vi "USBImageContinuousV1.9.vi"() -> ()   [LabVIEW 2019]
uses:
  atmcd32d.dll
panel:
  in  "Tab Control":T1(tab)
  out "Expected position on spectrometer (pixels):":dbl
  in  "Harmonic":dbl min=10.0 max=40.0
  out "l (nm)":dbl
  out "E (J)":dbl
  out "E (eV)":dbl
  out "Nearest Harmonic of 800nm":dbl
  out "Cursor Position (pixels)":dbl
  out "Distance to nearest harmonic of 800nm (pixels)":dbl
  in  "Grating:":u16(ring) items=["Shimadzu 30-006  "]
  in  "Laser:":u16(ring) items=["800nm  "]
  in  "Trigger":u32(ring) items=["Internal", "External"]
  in  "Exposure Time (secs)":sgl format="%.2f"
  out "Get Acquired Data":u32
  out "Start Acquisition":u32
  out "Detector X Pixels":i32
  out "Detector Y Pixels":i32
  out "Shut Down":u32
  out "Raw Image":i32[][](graph)
  out "Vertical Binned image":i32[](graph)
  out "Get Status":u32
  in  "Stop":bool
  in  "Save Image":bool
  out "Camera Status:":bool
  out "Last Image Saved:":string
  in  "Calibration Date":u16(ring) items=["first calibration - 7/31", "7/31-current"]
  out "Calibration Date: indicator:":u16(ring) items=["first calibration - 7/31", "7/31-current"]
  out "Status":u32
  out "Camera outputs":T2
  out "Camera inputs":T3
  in  "Correct for QE?":bool
  in  "IR Filter:":u16(ring)=1 items=["No filter", "100 nm Al", "200 nm Al", "250 nm Al", "500 nm Al"]
  out "Wavelength Graph (nm)":T4(graph)
  out "Energy Graph (eV)":cluster{"eV":dbl, "QE scaled count":dbl}[](graph)
  out "Harmonics Graph":cluster{dbl, "QE scaled count":dbl}[](graph)
  # "Acquisition Mode: Single Scan\nReadout Mode: Full Resolution Image"
  # "Return values"
  # "XUV Spectrometer Control VI"
  # "Status"
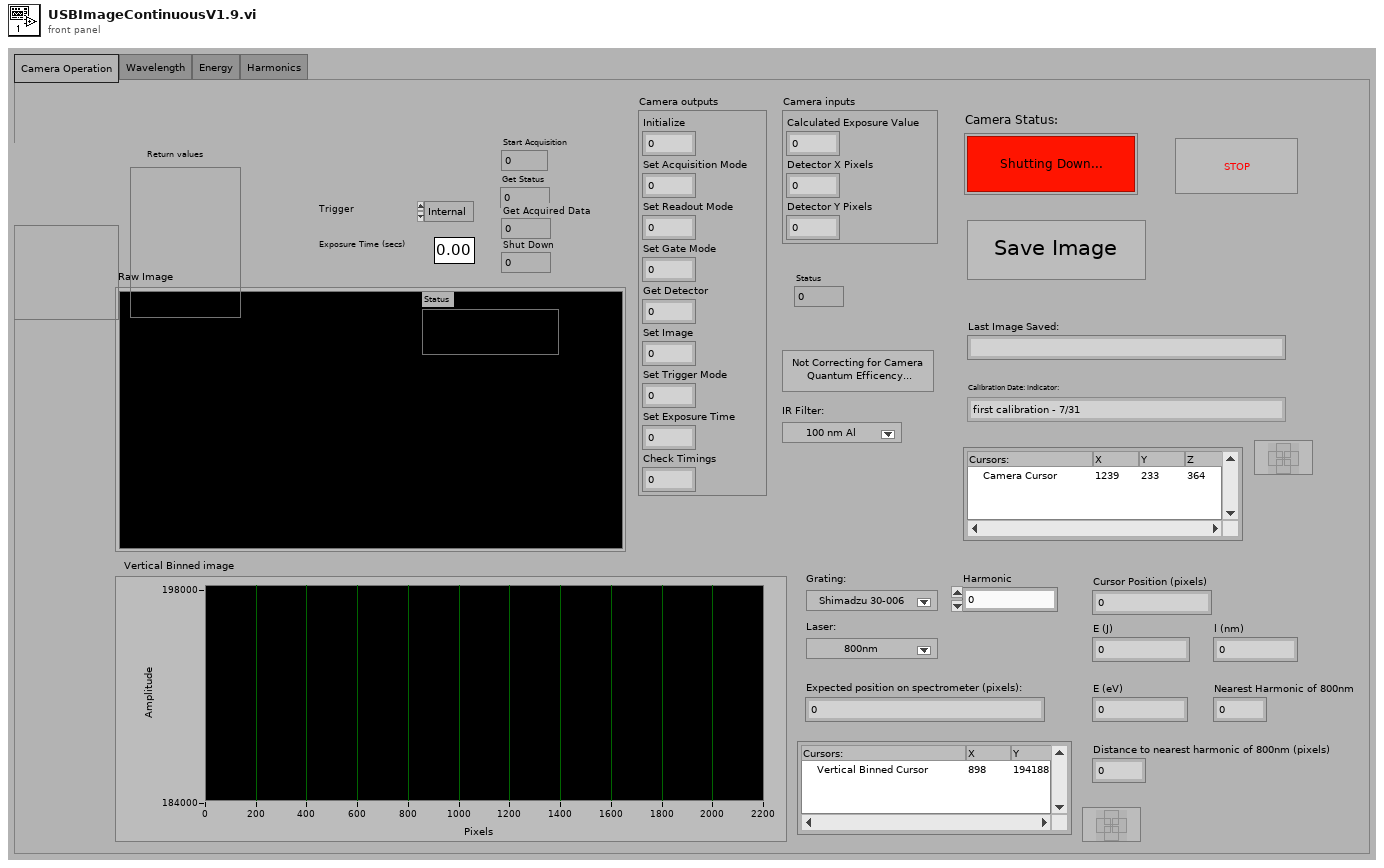
[diagram p1: front panel]
types:
  T1 = enum32{"Camera Operation", "Wavelength", "Energy", "Harmonics"}
  T2 = cluster{"Initialize":u32, "Set Acquisition Mode":u32, "Set Readout Mode":u32, "Set Gate Mode":u32, "Get Detector":u32, "Set Image":u32, "Set Trigger Mode":u32, "Set Exposure Time":u32, "Check Timings":u32}
  T3 = cluster{"Calculated Exposure Value":sgl, "Detector X Pixels":i32, "Detector Y Pixels":i32}
  T4 = cluster{"No prefix":dbl, "QE scaled count":dbl}[]
  T5 = cluster{"to shutdown":bool, "to get acquired data":bool, "to start acquisition":bool, "DRV_SUCCESS":i32}
  T6 = cluster{"No prefix":dbl, "filter scaled count":dbl}
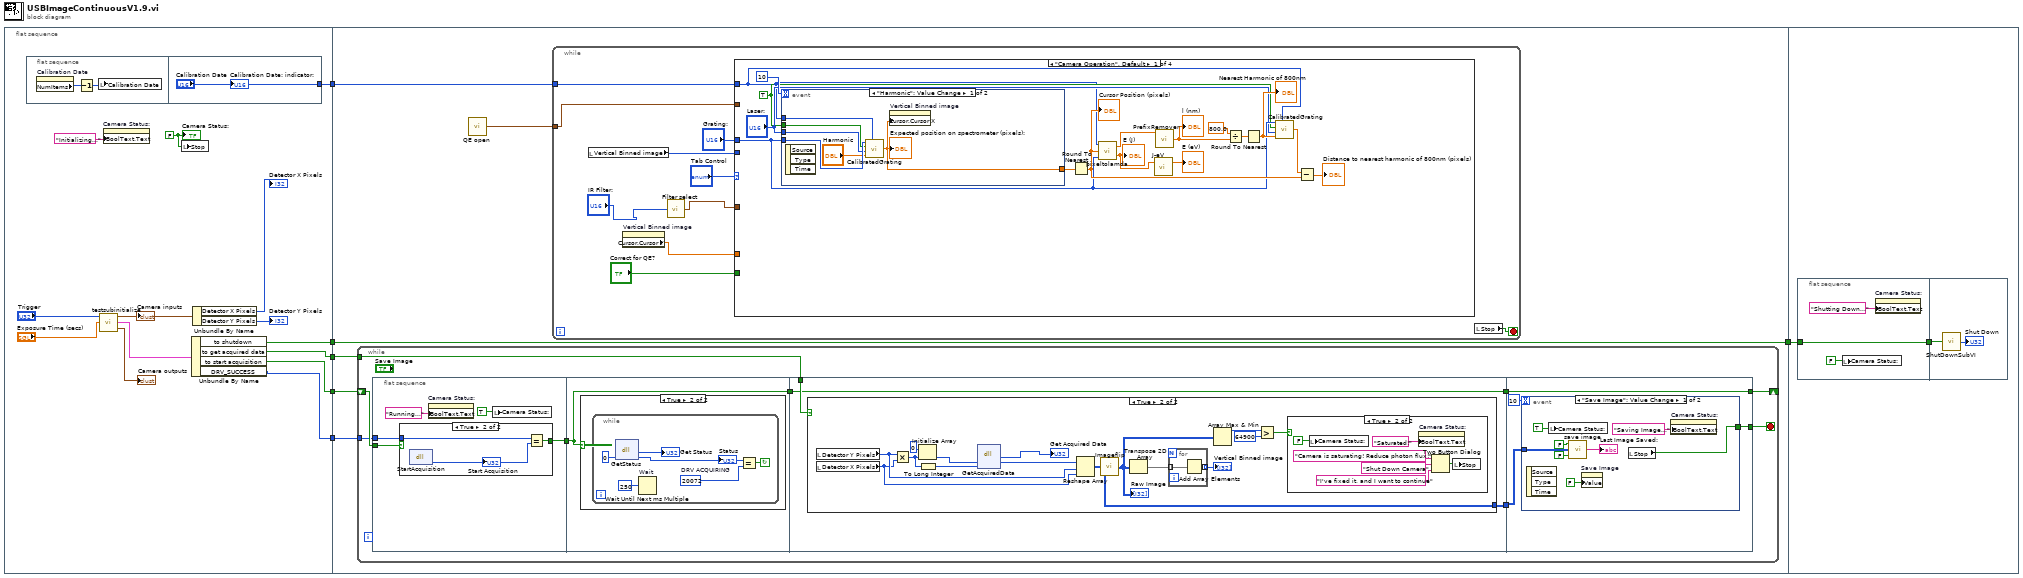
[diagram p0: block diagram]
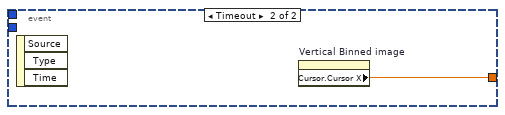
[diagram p2: hidden frame]
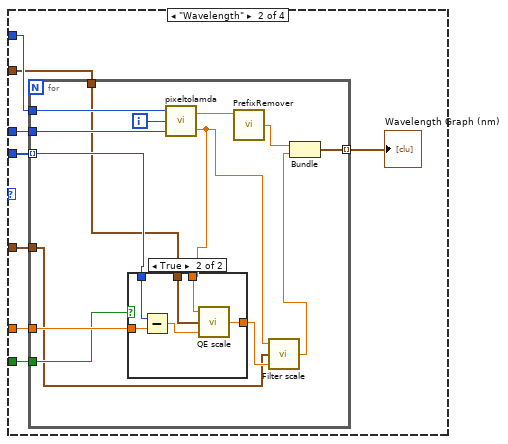
[diagram p3: hidden frame]
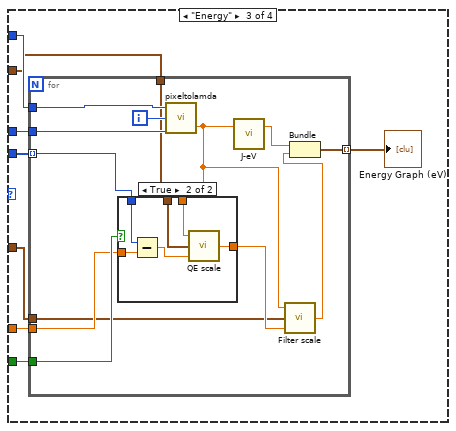
[diagram p5: hidden frame]
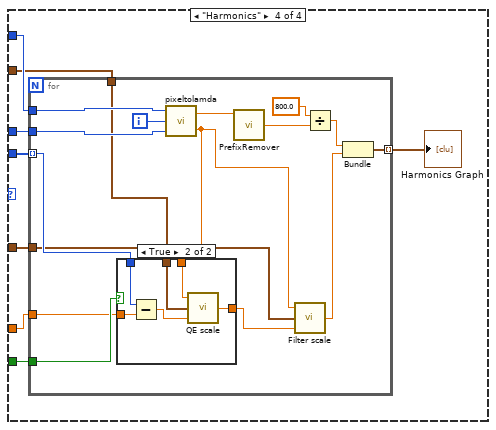
[diagram p7: hidden frame]
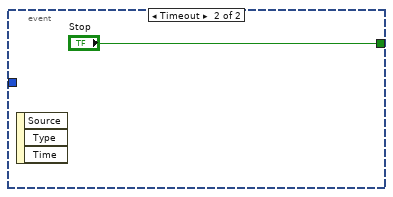
[diagram p13: hidden frame]
diagram:
  n1 = flat-sequence {
    tunnel: [w7] -> w5
    tunnel: [w8] -> w4
    tunnel: [w9] -> w3
    tunnel: [w10] -> w2
    tunnel: [w20] -> w1
    tunnel: [w26] -> w6
    tunnel: w5 -> [w29]
    tunnel: w4 -> [w28]
    tunnel: w3 -> [w27]
    tunnel: w2 -> [w26]
    tunnel: w1 -> [w25]
    tunnel: w6 -> [w215]
    frame #0 {
      w19 = FALSE ("Camera Status:")
      n2 = flat-sequence {
        tunnel: ["Calibration Date"] -> w20
        frame #0 {
          n3 = property on="Calibration Date" class="Ring (strict)"() -> ("NumItems"=w22:u32)  [unwired: 2 in, 2 out]
          n4 = Decrement(x=w22) -> (x-1=w21:u32)
          n5 = local write "Calibration Date"(w21) -> ()
        }
        frame #1 {
          "Calibration Date: indicator:" <- "Calibration Date"
        }
      }
      n6 = call "testsubinitialize.vi"("Exposure Time (secs)"="Exposure Time (secs)", "Trigger"="Trigger") -> ("Camera outputs"=→"Camera outputs":T2, "Camera status"=w17:T5, "Camera inputs"=w14:T3)  [unwired: 1 in]
      "Camera inputs" <- w14
      n7 = property on="Camera Status:" class="Bool (strict)"("BoolText.Text"="Initializing..." ("String")) -> ()  [unwired: 2 in, 2 out]
      n8 = local write "Stop"(w19) -> ()
      n9 = Unbundle By Name(w17) -> ("to shutdown"=w10:bool, "to get acquired data"=w9:bool, "to start acquisition"=w8:bool, "DRV_SUCCESS"=w7:i32)
      n10 = Unbundle By Name(w14) -> ("Detector X Pixels"=→"Detector X Pixels":i32, "Detector Y Pixels"=→"Detector Y Pixels":i32)
      "Camera Status:" <- w19
    }
    frame #1 {
      n11 = while {
        tunnel: w29 -> [w158]
        tunnel: w27 -> [w157]
        shift-right: [w153] -> _
        shift-left: w28 -> [w159]
        stop <- w151 stop-if-true
        n12 = flat-sequence {
          tunnel: w159 -> [w164]
          tunnel: w158 -> [w163]
          tunnel: [w162] -> w156
          tunnel: w156 -> [w169]
          tunnel: [w169] -> w155
          tunnel: w155 -> [w177]
          tunnel: w157 -> [w178]
          tunnel: [w177] -> w154
          tunnel: [w176] -> w152
          tunnel: w154 -> [w205]
          tunnel: w152 -> [w202]
          tunnel: [w203] -> w151
          tunnel: [w205] -> w153
          frame #0 {
            n13 = case shown="True" w164 {
              tunnel: [FALSE w168] -> w162
              tunnel: w163 -> [_ w167]
              frame False {
              }
              frame True {
                n14 = dll-call lib="atmcd32d.dll" fn="StartAcquisition" label="Call Library Function start acquisition"() -> (w166:u32)  [unwired: 3 in, 2 out]
                "Start Acquisition" <- w166
                n15 = Equal?(x=w167, y=w166) -> (x = y?=w168:bool)
              }
            }
            n16 = property on="Camera Status:" class="Bool (strict)"("BoolText.Text"="Running..." ("Boolean Text.Text")) -> ()  [unwired: 2 in, 2 out]
            n17 = local write "Camera Status:"(TRUE ("Camera Status:")) -> ()
          }
          frame #1 {
            n18 = case shown="True" w169 {
              frame False {
              }
              frame True {
                n19 = while {
                  stop <- w173 continue-if-true
                  w172 = u16 20072  # DRV ACQUIRING
                  n20 = dll-call lib="atmcd32d.dll" fn="GetStatus" label="Call Library Function GetAcquisitionStatus"(u16 0) -> (→"Get Status":u32, w171:u32)  [unwired: 3 in, 2 out]
                  "Status" <- w171
                  n21 = Wait Until Next ms Multiple "Wait"(millisecond multiple=u32 250) -> ()  [unwired: 1 out]
                  n22 = Equal?(x=w171, y=w172) -> (x = y?=w173:bool)
                }
              }
            }
          }
          frame #2 {
            n23 = case shown="True" w178 {
              tunnel: [_ w182] -> w176
              frame False {
              }
              frame True {
                n24 = local read "Detector Y Pixels"() -> (w188:i32)
                n25 = local read "Detector X Pixels"() -> (w184:i32)
                n26 = Multiply(x=w188, y=w184) -> (x*y=w190:i32)
                n27 = Initialize Array "Initialize Array"(0 ("Initial values in array"), w190) -> (w192:i32[])
                n28 = To Long Integer(number=w190) -> (32bit integer=w191:i32)
                n29 = dll-call lib="atmcd32d.dll" fn="GetAcquiredData" label="Call Library Function Get Acquired data"(w192, w191) -> (→"Get Acquired Data":u32, w189:i32[])  [unwired: 4 in, 2 out]
                n30 = Reshape Array(w189, w188, w184) -> (w182:i32[][])
                n31 = call "Imageflip.vi"("2D array"=w182) -> ("transposed array"=w180:i32[][])
                "Raw Image" <- w180
                n32 = Transpose 2D Array(2D array=w180) -> (transposed array=w187:i32[][])
                n33 = for {
                  tunnel: w187 -> [w201] mode=indexing
                  tunnel: [w200] -> w181 mode=indexing
                  n34 = Add Array Elements(numeric array=w201) -> (sum=w200:i32)
                }
                "Vertical Binned image" <- w181
                n35 = Array Max & Min(array=w180) -> (max value=w186:i32)  [unwired: 3 out]
                n36 = Greater?(x=w186, y=64900) -> (0:w185:bool)
                n37 = case shown="True" w185 {
                  frame False {
                  }
                  frame True {
                    n38 = local write "Camera Status:"(FALSE ("Camera Status:")) -> ()
                    n39 = property on="Camera Status:" class="Bool (strict)"("BoolText.Text"="Saturated!" ("Boolean Text.Text")) -> ()  [unwired: 2 in, 2 out]
                    n40 = Two Button Dialog(message="Camera is saturating! Reduce photon flux!", 1:"I've fixed it, and I want to continue" ("message"), 2:"Shut Down Camera" ("T button name (\"OK\")")) -> (T button?=w195:bool)
                    n41 = local write "Stop"(w195) -> ()
                  }
                }
              }
            }
          }
          frame #3 {
            n42 = event shown="[0] \"Save Image\": Value Change" {
              selector: _ -> [_ _]
              dyn-events: _ -> [_ _]
              timeout: 10 -> [_ _]
              tunnel: [w210 "Stop"] -> w203
              tunnel: w202 -> [w209 _]
              event "Save Image": Value Change {
                n43 = event-data() -> ()  [unwired: 1 in, 3 out]
                n44 = local write "Camera Status:"(TRUE ("Camera Status:")) -> ()
                n45 = call "save image.vi"("Start of pump/prove run?"=FALSE, "Image to save"=w209, "Pump/probe run?"=FALSE) -> ("Image file path"=→"Last Image Saved:":string)
                n46 = property on="Save Image" class="Bool (strict)"("Value"=FALSE ("Take image")) -> ()  [unwired: 2 in, 2 out]
                n47 = local read "Stop"() -> (w210:bool)
                n48 = property on="Camera Status:" class="Bool (strict)"("BoolText.Text"="Saving Image..." ("Boolean Text.Text")) -> ()  [unwired: 2 in, 2 out]
              }
              event Timeout {
                n49 = event-data() -> ()  [unwired: 1 in, 3 out]
              }
            }
          }
        }
      }
      n50 = call "QE open.vi"() -> ("QE data"=w24:cluster{"Numeric":dbl, dbl}[])
      n51 = while {
        tunnel: w25 -> [w35]
        tunnel: w24 -> [w34]
        stop <- w36 stop-if-true
        n52 = local read "Vertical Binned image"() -> (w38:i32[])
        n53 = property on="Vertical Binned image" class="WFGraph (strict)"() -> ("Cursor.Cursor Y"=w33:dbl)  [unwired: 2 in, 2 out]
        n54 = call "Filter select.vi"("Filter:"="IR Filter:") -> ("filter data"=w30:cluster{"Numeric":dbl, dbl}[])
        n55 = case shown="\"Camera Operation\", Default" "Tab Control" {
          tunnel: w38 -> [_ w70 w99 w127]
          tunnel: "Grating:" -> [w43 w69 w98 w126]
          tunnel: w35 -> [w40 w67 w96 w124]
          tunnel: w34 -> [_ w66 w93 w123]
          tunnel: w33 -> [_ w65 w94 w121]
          tunnel: "Correct for QE?" -> [_ w64 w95 w122]
          tunnel: w30 -> [_ w63 w92 w120]
          frame "Camera Operation", Default {
            w42 = TRUE
            n56 = event shown="[0] \"Harmonic\": Value Change" {
              selector: _ -> [_ _]
              dyn-events: _ -> [_ _]
              timeout: 10 -> [_ _]
              tunnel: [w57 w62] -> w44
              tunnel: w43 -> [w61 _]
              tunnel: w42 -> [w60 _]
              tunnel: "Laser:" -> [w59 _]
              tunnel: w40 -> [w58 _]
              event "Harmonic": Value Change {
                n57 = event-data() -> ()  [unwired: 1 in, 3 out]
                n58 = call "CalibratedGrating.vi"("Grating:"=w61, "Subvi?"=w60, "Laser:"=w59, "Harmonic"="Harmonic", "Caibration Date"=w58) -> ("Position on spectrometer (pixels):"=w57:dbl)
                "Expected position on spectrometer (pixels):" <- w57
                n59 = property on="Vertical Binned image" class="WFGraph (strict)"("Cursor.Cursor X"=w57) -> ()  [unwired: 2 in, 2 out]
              }
              event Timeout {
                n60 = event-data() -> ()  [unwired: 1 in, 3 out]
                n61 = property on="Vertical Binned image" class="WFGraph (strict)"() -> ("Cursor.Cursor X"=w62:dbl)  [unwired: 2 in, 2 out]
              }
            }
            n62 = Round To Nearest(number=w44) -> (nearest integer value=w49:dbl)
            "Cursor Position (pixels)" <- w49
            n63 = call "pixeltolamda.vi"("Grating:"=w43, "Pixel Postion"=w49, "Caibration Date"=w40) -> ("E (J)"=w51:dbl, "lamda (m)"=w55:dbl)
            "E (J)" <- w51
            n64 = call "J-eV.vi"("J"=w51) -> ("eV"=→"E (eV)":dbl)  [unwired: 1 in, 1 out]
            n65 = call "PrefixRemover.vi"("Nano"=w55) -> ("No prefix"=w52:dbl)  [unwired: 3 in]
            "l (nm)" <- w52
            n66 = Divide(x=800.0, y=w52) -> (x/y=w54:dbl)
            n67 = Round To Nearest(number=w54) -> (nearest integer value=w48:dbl)
            "Nearest Harmonic of 800nm" <- w48
            n68 = call "CalibratedGrating.vi"("Grating:"=w43, "Subvi?"=w42, "Laser:"="Laser:", "Harmonic"=w48, "Caibration Date"=w40) -> ("Position on spectrometer (pixels):"=w47:dbl)
            n69 = Subtract(x=w47, y=w49) -> (x-y=→"Distance to nearest harmonic of 800nm (pixels)":dbl)
          }
          frame "Wavelength" {
            n70 = for {
              tunnel: w70 -> [w78] mode=indexing
              tunnel: w69 -> [w82]
              tunnel: [w80] -> w68 mode=indexing
              tunnel: w67 -> [w79]
              tunnel: w66 -> [w77]
              tunnel: w65 -> [w76]
              tunnel: w64 -> [w75]
              tunnel: w63 -> [w71]
              i -> [w81]
              n71 = call "pixeltolamda.vi"("Grating:"=w82, "Pixel Postion"=w81, "Caibration Date"=w79) -> ("E (J)"=w72:dbl, "lamda (m)"=w83:dbl)
              n72 = case shown="True" w75 {
                tunnel: w76 -> [_ w91]
                tunnel: w78 -> [w85 w90]
                tunnel: w77 -> [_ w88]
                tunnel: w72 -> [_ w87]
                tunnel: [w85 w86] -> w74
                frame False {
                }
                frame True {
                  n73 = Subtract(x=w90, y=w91) -> (x-y=w89:dbl)
                  n74 = call "QE scale.vi"("Raw Photon Count"=w89, "QE data"=w88, "Energy (J)"=w87) -> ("QE scaled count"=w86:dbl)
                }
              }
              n75 = call "PrefixRemover.vi"("Nano"=w83) -> ("No prefix"=w84:dbl)  [unwired: 3 in]
              n76 = call "Filter scale.vi"("Raw Photon Count"=w74, "filter data"=w71, "Energy (J)"=w72) -> ("filter scaled count"=w73:dbl)
              n77 = Bundle("No prefix"=w84, "filter scaled count"=w73) -> (w80:T6)  [unwired: 1 in]
            }
            "Wavelength Graph (nm)" <- w68
          }
          frame "Energy" {
            n78 = for {
              tunnel: w99 -> [w107] mode=indexing
              tunnel: w98 -> [w111]
              tunnel: [w109] -> w97 mode=indexing
              tunnel: w96 -> [w108]
              tunnel: w95 -> [w106]
              tunnel: w94 -> [w105]
              tunnel: w93 -> [w104]
              tunnel: w92 -> [w100]
              i -> [w112]
              n79 = call "pixeltolamda.vi"("Grating:"=w111, "Pixel Postion"=w112, "Caibration Date"=w108) -> ("E (J)"=w102:dbl)  [unwired: 1 out]
              n80 = case shown="True" w106 {
                tunnel: w105 -> [_ w119]
                tunnel: w107 -> [w113 w118]
                tunnel: w104 -> [_ w116]
                tunnel: w102 -> [_ w115]
                tunnel: [w113 w114] -> w103
                frame False {
                }
                frame True {
                  n81 = Subtract(x=w118, y=w119) -> (x-y=w117:dbl)
                  n82 = call "QE scale.vi"("Raw Photon Count"=w117, "QE data"=w116, "Energy (J)"=w115) -> ("QE scaled count"=w114:dbl)
                }
              }
              n83 = call "J-eV.vi"("J"=w102) -> ("eV"=w110:dbl)  [unwired: 1 in, 1 out]
              n84 = call "Filter scale.vi"("Raw Photon Count"=w103, "filter data"=w100, "Energy (J)"=w102) -> ("filter scaled count"=w101:dbl)
              n85 = Bundle("eV"=w110, "filter scaled count"=w101) -> (w109:cluster{"eV":dbl, "filter scaled count":dbl})  [unwired: 1 in]
            }
            "Energy Graph (eV)" <- w97
          }
          frame "Harmonics" {
            n86 = for {
              tunnel: w127 -> [w134] mode=indexing
              tunnel: w126 -> [w142]
              tunnel: [w140] -> w125 mode=indexing
              tunnel: w124 -> [w136]
              tunnel: w123 -> [w135]
              tunnel: w122 -> [w133]
              tunnel: w121 -> [w132]
              tunnel: w120 -> [w128]
              i -> [w141]
              n87 = call "pixeltolamda.vi"("Grating:"=w142, "Pixel Postion"=w141, "Caibration Date"=w136) -> ("E (J)"=w129:dbl, "lamda (m)"=w143:dbl)
              n88 = case shown="True" w133 {
                tunnel: w132 -> [_ w150]
                tunnel: w134 -> [w144 w149]
                tunnel: w135 -> [_ w147]
                tunnel: w129 -> [_ w146]
                tunnel: [w144 w145] -> w131
                frame False {
                }
                frame True {
                  n89 = Subtract(x=w149, y=w150) -> (x-y=w148:dbl)
                  n90 = call "QE scale.vi"("Raw Photon Count"=w148, "QE data"=w147, "Energy (J)"=w146) -> ("QE scaled count"=w145:dbl)
                }
              }
              n91 = call "PrefixRemover.vi"("Nano"=w143) -> ("No prefix"=w138:dbl)  [unwired: 3 in]
              n92 = call "Filter scale.vi"("Raw Photon Count"=w131, "filter data"=w128, "Energy (J)"=w129) -> ("filter scaled count"=w130:dbl)
              n93 = Divide(x=800.0, y=w138) -> (x/y=w137:dbl)
              n94 = Bundle(w137, "filter scaled count"=w130) -> (w140:cluster{dbl, "filter scaled count":dbl})  [unwired: 1 in]
            }
            "Harmonics Graph" <- w125
          }
        }
        n95 = local read "Stop"() -> (w36:bool)
      }
    }
    frame #2 {
      n96 = flat-sequence {
        tunnel: w215 -> [w219]
        tunnel: [w219] -> w216
        tunnel: w216 -> [w221]
        frame #0 {
          n97 = local write "Camera Status:"(FALSE ("Camera Status:")) -> ()
          n98 = property on="Camera Status:" class="Bool (strict)"("BoolText.Text"="Shutting Down..." ("Boolean Text.Text")) -> ()  [unwired: 2 in, 2 out]
        }
        frame #1 {
          n99 = call "ShutDownSubVI.vi"("shutdown"=w221) -> ("Shut Down"=→"Shut Down":u32)
        }
      }
    }
  }
